vi "OAT_Campbell Diagram_Indics to EU.vi"(9 "y scale":cluster{"offset":dbl, "multiplier":dbl} {"multiplier" format="%.2f"; "offset" format="%.2f"}, 10 "x scale":cluster{"offset":dbl, "multiplier":dbl} {"multiplier" format="%.2f"; "offset" format="%.2f"}, 11 "indices":i32[](array[numeric])) -> (2 "y [EU]":dbl format="%.2f", 3 "x [EU]":dbl format="%.2f")   [LabVIEW 2017]
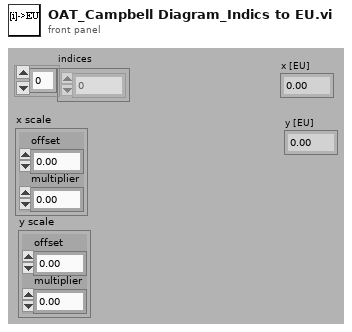
[diagram p1: front panel]
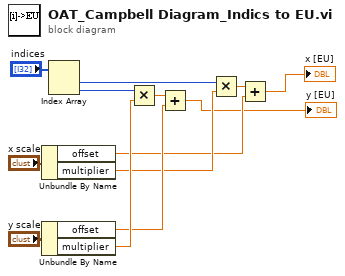
[diagram p0: block diagram]
diagram:
  n1 = Unbundle By Name("x scale") -> ("offset"=w3:dbl, "multiplier"=w5:dbl)
  n2 = Unbundle By Name("y scale") -> ("offset"=w7:dbl, "multiplier"=w8:dbl)
  n3 = Index Array(array="indices") -> (element #1=w6:i32, element #2=w10:i32)  [unwired: 2 in]
  n4 = Multiply(x=w10, y=w8) -> (x*y=w9:dbl)
  n5 = Add(x=w9, y=w7) -> (x+y=→"y [EU]":dbl)
  n6 = Multiply(x=w6, y=w5) -> (x*y=w4:dbl)
  n7 = Add(x=w4, y=w3) -> (x+y=→"x [EU]":dbl)
